vi "niFPGA FFT Permute Inputs.vi"(0 "input index":u16, 5 "input valid":bool, 7 "K - 16":i8) -> (4 "permuted index":u16, 6 "write input to A":bool, 8 "write input to B":bool)   [LabVIEW 2017]
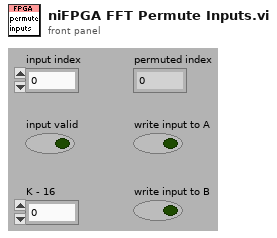
[diagram p1: front panel]
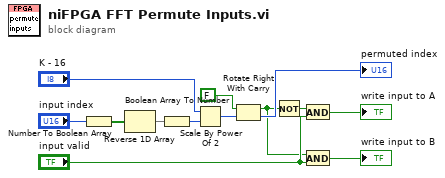
[diagram p0: block diagram]
diagram:
  n1 = Number To Boolean Array(number="input index") -> (Boolean array=w5:bool[])
  n2 = Reverse 1D Array(array=w5) -> (reversed array=w3:bool[])
  n3 = Boolean Array To Number(Boolean array=w3) -> (number=w6:u16)
  n4 = Scale By Power Of 2(n="K - 16", x=w6) -> (x*2^n=w7:u16)
  n5 = Rotate Right With Carry(2:w7, 3:FALSE ("carry")) -> (0:→"permuted index":u16, 1:w9:bool)
  n6 = Not(x=w9) -> (.not. x?=w4:bool)
  n7 = And(x=w4, y="input valid") -> (x .and. y?=→"write input to A":bool)
  n8 = And(x=w9, y="input valid") -> (x .and. y?=→"write input to B":bool)
